vi "Read ADU.vi"(8 "error in (no error)":errorcluster, 11 "MB_Master in":refnum<class "MB_Master.lvclass">) -> (0 "error out":errorcluster, 2 "MB_ADU":refnum<class "MB_ADU.lvclass">, 3 "MB_Master out":refnum<class "MB_Master.lvclass">)   [LabVIEW 2023, in "Jiaxin_Stepper_Controller.lvlib" / "MB Master.lvlib" / "MB_Master.lvclass"]
uses:
  MB_Master.lvclass
  MB_ADU/MB_ADU.lvclass
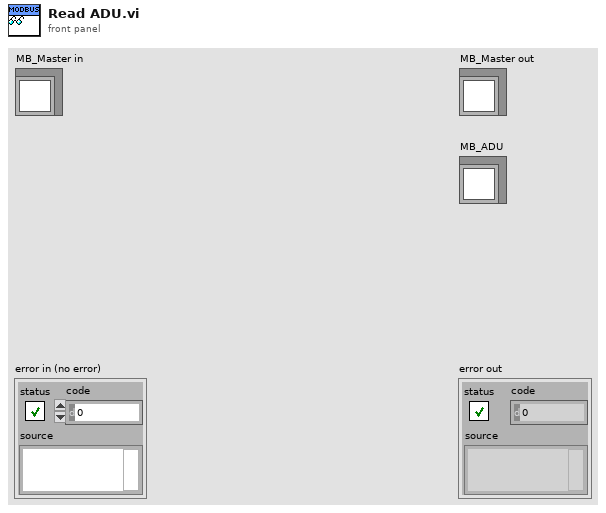
[diagram p1: front panel]
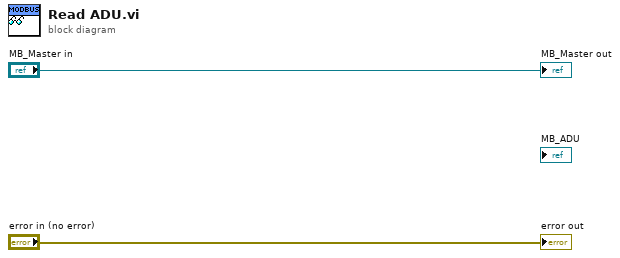
[diagram p0: block diagram]
diagram:
  "error out" <- "error in (no error)"
  "MB_Master out" <- "MB_Master in"
